vi "Index.vi"(9 "Messbereich":u16, 11 "Komponente":u16) -> (0 "Index Analysator":u16, 1 "Index Komponente":u16, 3 "Index Lin":u16, 4 "Komponente (Text)":string)   [LabVIEW 2020, in "Erweiterte Konfig.lvlib" / "CG-Check Konfig.lvlib"]
uses:
  CG-Check Konfig.lvlib
  FT-IR/FGV FT-IR Gasliste Aktionen.ctl
  FT-IR/FT-IR.lvlib
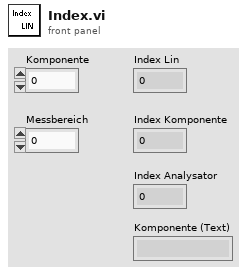
[diagram p1: front panel]
types:
  T1 = typedef "FT-IR.lvlib/FGV FT-IR Gasliste Aktionen.ctl" = enum16{"lesen", "Gasliste FT-IR", "Gasliste ausgelesen", "laden", "speichern", "löschen"}
  T2 = typedef "String - Ausgabefeld.ctl" = string
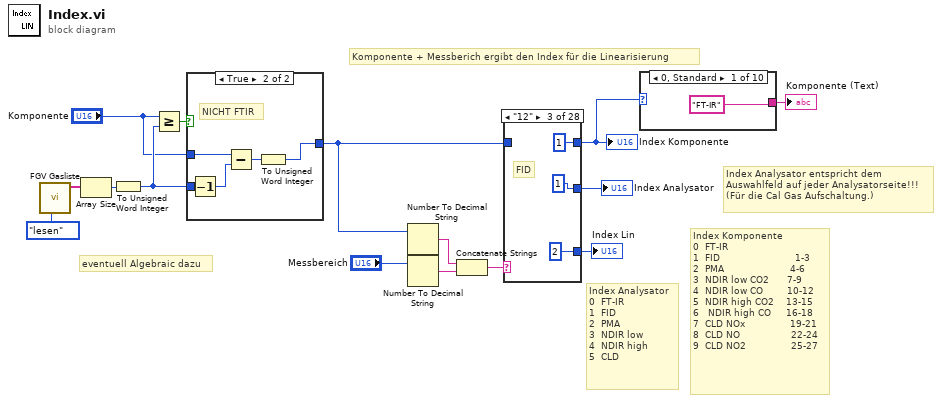
[diagram p0: block diagram]
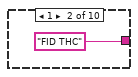
[diagram p2: hidden frame]
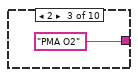
[diagram p3: hidden frame]
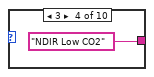
[diagram p4: hidden frame]
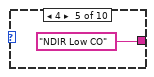
[diagram p5: hidden frame]
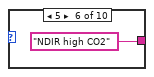
[diagram p6: hidden frame]
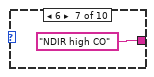
[diagram p7: hidden frame]
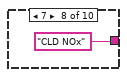
[diagram p8: hidden frame]
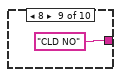
[diagram p9: hidden frame]
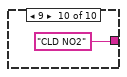
[diagram p10: hidden frame]
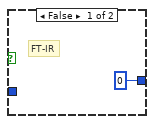
[diagram p11: hidden frame]
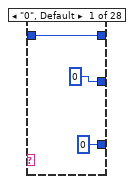
[diagram p12: hidden frame]
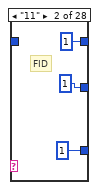
[diagram p13: hidden frame]
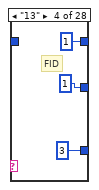
[diagram p14: hidden frame]
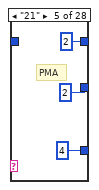
[diagram p15: hidden frame]
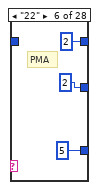
[diagram p16: hidden frame]
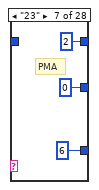
[diagram p17: hidden frame]
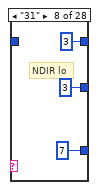
[diagram p18: hidden frame]
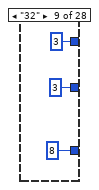
[diagram p19: hidden frame]
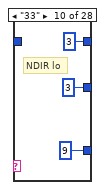
[diagram p20: hidden frame]
diagram:
  # "Index Analysator\n0  FT-IR\n1  FID\n2  PMA  \n3  NDIR low\n4  NDIR high \n5  CLD"
  # "Index Analysator entspricht dem \nAuswahlfeld auf jeder Analysatorseite!!!\n(Für die Cal Gas Aufschaltung.)"
  # "eventuell Algebraic dazu"
  # "Index Komponente\n0  FT-IR\n1  FID                         1-3\n2  PMA                      4-6\n3  NDIR low CO2      7-9\n4  NDIR low CO        10-12\n5  NDIR high CO2    13-15\n6   NDIR high CO     16-18\n7  CLD NOx               19-21\n8  CLD NO                 22-24\n9  CLD NO2               25-27"
  # "Komponente + Messberich ergibt den Index für die Linearisierung"
  n1 = call "FGV Gasliste.vi"("Aktionen"=FGV_FT-IR_Gasliste_Aktionen."lesen") -> ("Aktuelle Gasliste FT-IR"=w11:T2[])  [unwired: 8 in, 2 out]
  n2 = Array Size(array=w11) -> (size(s)=w9:i32)
  n3 = To Unsigned Word Integer(number=w9) -> (unsigned 16bit integer=w8:u16)
  n4 = Greater Or Equal?(x="Komponente", y=w8) -> (x >= y?=w10:bool)
  n5 = case shown="True" w10 {
    tunnel: "Komponente" -> [_ w21]
    tunnel: w8 -> [_ w20]
    tunnel: [u16 0 w17] -> w5
    frame False {
      # "FT-IR"
    }
    frame True {
      # "NICHT FTIR"
      n6 = Decrement(x=w20) -> (x-1=w19:u16)
      n7 = Subtract(x=w21, y=w19) -> (x-y=w18:u16)
      n8 = To Unsigned Word Integer(number=w18) -> (unsigned 16bit integer=w17:u16)
    }
  }
  n9 = Number To Decimal String(number=w5) -> (decimal integer string=w15:string)  [unwired: 1 in]
  n10 = Number To Decimal String(number="Messbereich") -> (decimal integer string=w14:string)  [unwired: 1 in]
  n11 = Concatenate Strings(w15, w14) -> (w4:string)
  n12 = case shown="\"12\"" w4 {
    tunnel: [u16 0 u16 1 u16 2 u16 3 u16 4 u16 5 u16 6 u16 7 u16 8 u16 9 u16 10 u16 11 u16 12 u16 13 u16 14 u16 15 u16 16 u16 17 u16 18 u16 19 u16 20 u16 21 u16 22 u16 23 u16 24 u16 25 u16 26 u16 27] -> w12
    tunnel: w5 -> [w23 _ _ _ _ _ _ _ _ _ _ _ _ _ _ _ _ _ _ _ _ _ _ _ _ _ _ _]
    tunnel: [w23 u16 1 u16 1 u16 1 u16 2 u16 2 u16 2 u16 3 u16 3 u16 3 u16 4 u16 4 u16 4 u16 5 u16 5 u16 5 u16 6 u16 6 u16 6 u16 7 u16 7 u16 7 u16 8 u16 8 u16 8 u16 9 u16 9 u16 9] -> w2
    tunnel: [u16 0 u16 1 u16 1 u16 1 u16 2 u16 2 u16 0 u16 3 u16 3 u16 3 u16 3 u16 3 u16 3 u16 4 u16 4 u16 4 u16 4 u16 4 u16 4 u16 5 u16 5 u16 5 u16 5 u16 5 u16 5 u16 5 u16 5 u16 5] -> w3
    frame "0", Default {
    }
    frame "11" {
      # "FID"
    }
    frame "12" {
      # "FID"
    }
    frame "13" {
      # "FID"
    }
    frame "21" {
      # "PMA"
    }
    frame "22" {
      # "PMA"
    }
    frame "23" {
      # "PMA"
    }
    frame "31" {
      # "NDIR lo"
    }
    frame "32" {
    }
    frame "33" {
      # "NDIR lo"
    }
    frame "41" {
      # "NDIR lo"
    }
    frame "42" {
      # "NDIR lo"
    }
    frame "43" {
      # "NDIR lo"
    }
    frame "51" {
      # "NDIR hi"
    }
    frame "52" {
      # "NDIR hi"
    }
    frame "53" {
      # "NDIR hi"
    }
    frame "61" {
      # "NDIR hi"
    }
    frame "62" {
      # "NDIR hi"
    }
    frame "63" {
      # "NDIR hi"
    }
    frame "71" {
      # "NOx"
    }
    frame "72" {
      # "NOx"
    }
    frame "73" {
      # "NOx"
    }
    frame "81" {
      # "NO"
    }
    frame "82" {
      # "NO"
    }
    frame "83" {
      # "NO"
    }
    frame "91" {
      # "NO2"
    }
    frame "92" {
      # "NO2"
    }
    frame "93" {
      # "NO2"
    }
  }
  "Index Lin" <- w12
  "Index Komponente" <- w2
  "Index Analysator" <- w3
  n13 = case shown="0, Standard" w2 {
    tunnel: ["FT-IR" ("Titelzeile") "FID THC" ("Titelzeile") "PMA O2" ("Titelzeile") "NDIR Low CO2" ("Titelzeile") "NDIR Low CO" ("Titelzeile") "NDIR high CO2" ("Titelzeile") "NDIR high CO" ("Titelzeile") "CLD NOx" ("Titelzeile") "CLD NO" ("Titelzeile") "CLD NO2" ("Titelzeile")] -> w1
    frame 0, Default {
    }
    frame 1 {
    }
    frame 2 {
    }
    frame 3 {
    }
    frame 4 {
    }
    frame 5 {
    }
    frame 6 {
    }
    frame 7 {
    }
    frame 8 {
    }
    frame 9 {
    }
  }
  "Komponente (Text)" <- w1
